vi "Protocol Read to CRLF.vi"(8 "error in":errorcluster, 9 "timeout":i32=10000, 10 "bytes to read":i32, 11 "protocol layer in":refnum<class "Network Protocol.lvclass">) -> (0 "error out":errorcluster, 1 "timed out?":bool, 2 "data":u8[](array[numeric]), 3 "protocol layer out":refnum<class "Network Protocol.lvclass">)   [LabVIEW 2013, in "Network Protocol.lvclass"]
doc: "This provides an interface for reading from a network bus."
uses:
  Network Protocol.lvclass
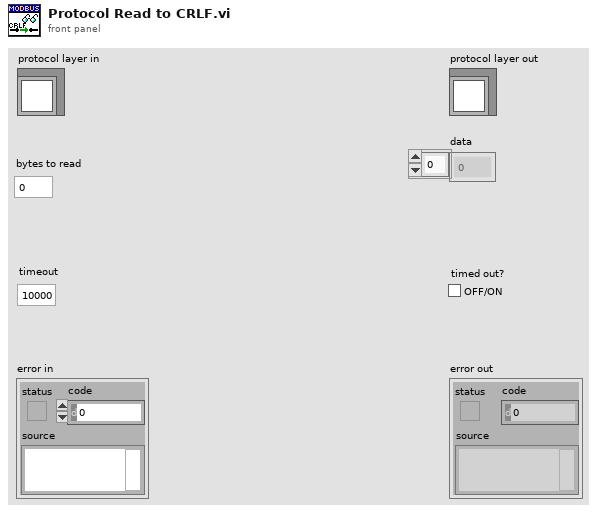
[diagram p1: front panel]
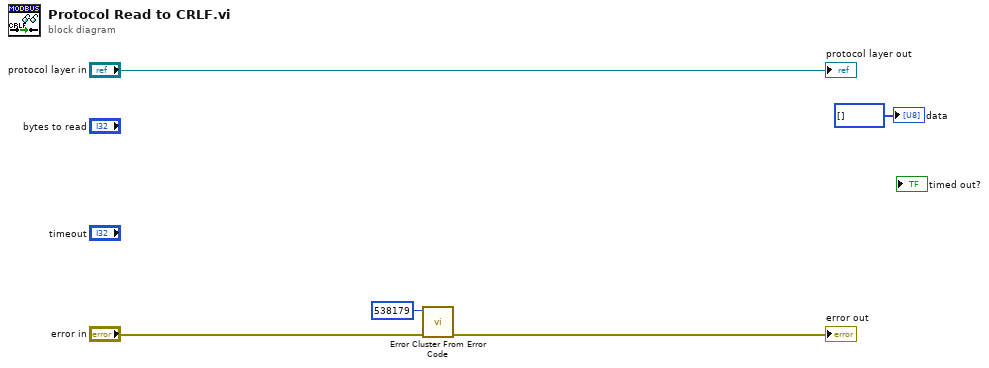
[diagram p0: block diagram]
diagram:
  n1 = call <vilib>:"Error Cluster From Error Code.vi"("error in (no error)"="error in", "error code (0)"=538179) -> ("error out"=→"error out":errorcluster)  [unwired: 7 in]
  "protocol layer out" <- "protocol layer in"
  "data" <- u8[] [] ("data")
